vi "Zusatzinformationen auslesen(SubVI).vi"(0 "Zusatzinformationen":string, 14 "Format+Namen":string) -> (20 "1":dbl, 21 "2":dbl, 22 "3":dbl, 23 "4":dbl, 24 "5":dbl, 25 "6":dbl, 26 "7":dbl, 27 "8":dbl)   [LabVIEW 2010]
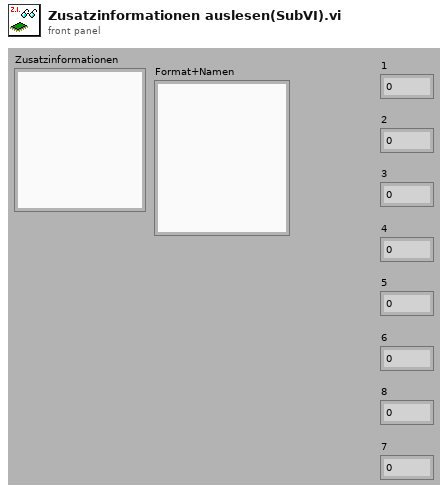
[diagram p1: front panel]
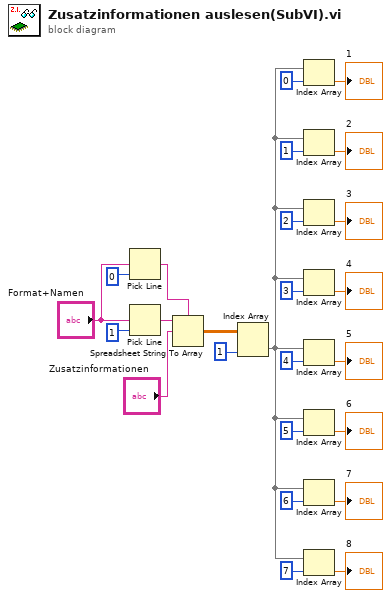
[diagram p0: block diagram]
diagram:
  n1 = Pick Line(multi-line string="Format+Namen", line index=0 ("Zeilenindex")) -> (output string=w20:string)  [unwired: 1 in]
  n2 = Pick Line(multi-line string="Format+Namen", line index=1 ("Zeilenindex")) -> (output string=w19:string)  [unwired: 1 in]
  n3 = Spreadsheet String To Array(delimiter (Tab)=w20, format string=w19, spreadsheet string="Zusatzinformationen") -> (array=w22:dbl[][])  [unwired: 1 in]
  n4 = Index Array(array=w22, index (col)=1 ("Deaktivierter Index (Spalte)")) -> (element=w17:dbl[])  [unwired: 1 in]
  n5 = Index Array(array=w17, index=0 ("Index")) -> (element=→"1":dbl)
  n6 = Index Array(array=w17, index=1 ("Index")) -> (element=→"2":dbl)
  n7 = Index Array(array=w17, index=2 ("Index")) -> (element=→"3":dbl)
  n8 = Index Array(array=w17, index=3 ("Index")) -> (element=→"4":dbl)
  n9 = Index Array(array=w17, index=4 ("Index")) -> (element=→"5":dbl)
  n10 = Index Array(array=w17, index=5 ("Index")) -> (element=→"6":dbl)
  n11 = Index Array(array=w17, index=6 ("Index")) -> (element=→"7":dbl)
  n12 = Index Array(array=w17, index=7 ("Index")) -> (element=→"8":dbl)
